vi "教導.vi"() -> ()   [LabVIEW 2015]
panel:
  out "密碼正確":bool
  in  "02A-5 Home Flag":bool
  out "Home TimeOut 2":dbl format="%.2f"
  in  "Home TimeOut In 2":dbl=30000.0 format="%#_13g"
  out "單軸復歸進行 2":bool
  out "Home TimeOut":dbl format="%.2f"
  in  "Home TimeOut In":dbl=30000.0 format="%#_13g"
  out "單軸復歸進行":bool
  out "存檔":bool
  in  "Recipe Ring":u8(ring) items=["abc.ini", "LeTV.ini", "小米.ini"]
  in  "Jog_Speed":i32
  in  "Jog Ring":u16(ring) items=["距離移動", "連續移動"]
  in  "Step Ring":u16(ring) items=["0.001 mm", "0.01 mm", "0.1 mm", "1 mm"]
  out "Tab 機構部件":T1(tab)
  out "Tab 設定位置入Tray站":enum32{"取Tray馬達", "收Tray馬達"}(tab) caption="Tab 設定位置"
  in  "入Tray站_分Tray位":dbl=100.0 caption="分Tray位" min=100.0 max=115.0
  in  "入Tray站_取Tray位":dbl=120.0 caption="取Tray位" min=115.0 max=125.0
  in  "入Tray站_待Tray位":dbl caption="待Tray位" min=0.0 max=5.0
  in  "Save_入Tray站_取Tray馬達":bool
  in  "入Tray站_收Tray位":dbl caption="收Tray上升距離" min=0.0 max=40.0
  in  "Save_入Tray站_收Tray馬達":bool
  in  "JOG_Up":bool
  in  "JOG_Down":bool
  in  "馬達選擇":u32(ring) items=["取Tray馬達", "收Tray馬達"]
  out "Tab 設定位置入料站":enum32{"等待位", "取料位", "放料位", "拍照位"}(tab) caption="Tab 設定位置"
  in  "JOG_Up 2":bool
  in  "JOG_Down 2":bool
  in  "JOG_R 2":bool
  in  "JOG_L 2":bool
  in  "點位選擇02A":u32(ring) items=["等待位", "取料位", "放料位", "拍照位"]
  in  "小Y":bool caption="Y¶b(¤pY)"
  in  "JOG_Down 2b 2":bool
  in  "JOG_Up 2b 2":bool
  in  "JOG_C02-":bool
  in  "JOG_C02+":bool
  in  "JOG_C01-":bool
  in  "JOG_C01+":bool
  in  "JOG_R 2b2":bool
  in  "JOG_L 2b2":bool
  out "Tab 設定位置入料站02B":enum32{"取料位", "安全位", "NG位", "拍照位", "放料位"}(tab) caption="Tab 設定位置"
  in  "JOG_Up 2b":bool
  in  "JOG_Down 2b":bool
  in  "JOG_R 2b1":bool
  in  "JOG_L 2b1":bool
  in  "點位選擇02B":u32(ring) items=["取料位", "安全位", "NG位", "拍照位", "放料位", "", ""]
  out "Tab 設定位置Ag站":enum32{"清潔位"}(tab) caption="Tab 設定位置"
  in  "JOG_Up 4":bool
  in  "JOG_Down 4":bool
  in  "JOG_R 4":bool
  in  "JOG_L 4":bool
  in  "點位選擇04":u32(ring) items=["清潔位", "取料位", "放料位"]
  out "Tab 設定位置UV站":enum32{"清潔位", "點膠位"}(tab) caption="Tab 設定位置"
  in  "JOG_Up 5":bool
  in  "JOG_Down 5":bool
  in  "JOG_R 5":bool
  in  "JOG_L 5":bool
  in  "點位選擇05":u32(ring) items=["清潔位", "點膠位", "放料位"]
  in  "JOG_旋轉 +":bool
  in  "JOG_旋轉 -":bool
  out "Tab 設定位置\n出料站":enum32{"等待位", "取料位", "放料位"}(tab) caption="Tab 設定位置"
  in  "JOG_Up 9":bool
  in  "JOG_Down 9":bool
  in  "JOG_R 9":bool
  in  "JOG_L 9":bool
  in  "點位選擇09":u32(ring) items=["等待位", "取料位", "放料位"]
  out "Tab 設定位置出Tray站":enum32{"取Tray馬達", "收Tray馬達"}(tab) caption="Tab 設定位置"
  in  "JOG_Up 10":bool
  in  "JOG_Down 10":bool
  out "出Tray站_馬達位置":dbl caption="馬達位置"
  in  "馬達選擇10":u32(ring) items=["取Tray馬達", "收Tray馬達"]
  in  "機構部件":T2(ring)
  in  "Exit":bool
  # "教導"
  # "馬達移動"
  # "mm/s"
  # "現在位置(mm)"
  # "JOG"
  # "設定位置(mm)"
  # "設定位置(mm)"
  # "現在位置(mm)"
  # "JOG"
  # "設定位置(mm)"
  # "設定位置(mm)"
  # "設定位置(mm)"
  # "設定位置(mm)"
  # "現在位置(mm)"
  # "JOG"
  # "設定位置(mm)"
  # "設定位置(mm)"
  # "設定位置(mm)"
  # "設定位置(mm)"
  # "設定位置(mm)"
  # "現在位置(mm)"
  # "JOG"
  # "設定位置(mm)"
  # "現在位置(mm)"
  # "JOG"
  # "設定位置(mm)"
  # "設定位置(mm)"
  # "現在位置(mm)"
  # "JOG"
  # "設定位置(mm)"
  # "設定位置(mm)"
  # "設定位置(mm)"
  # "現在位置(mm)"
  # "JOG"
  # "設定位置(mm)"
  # "設定位置(mm)"
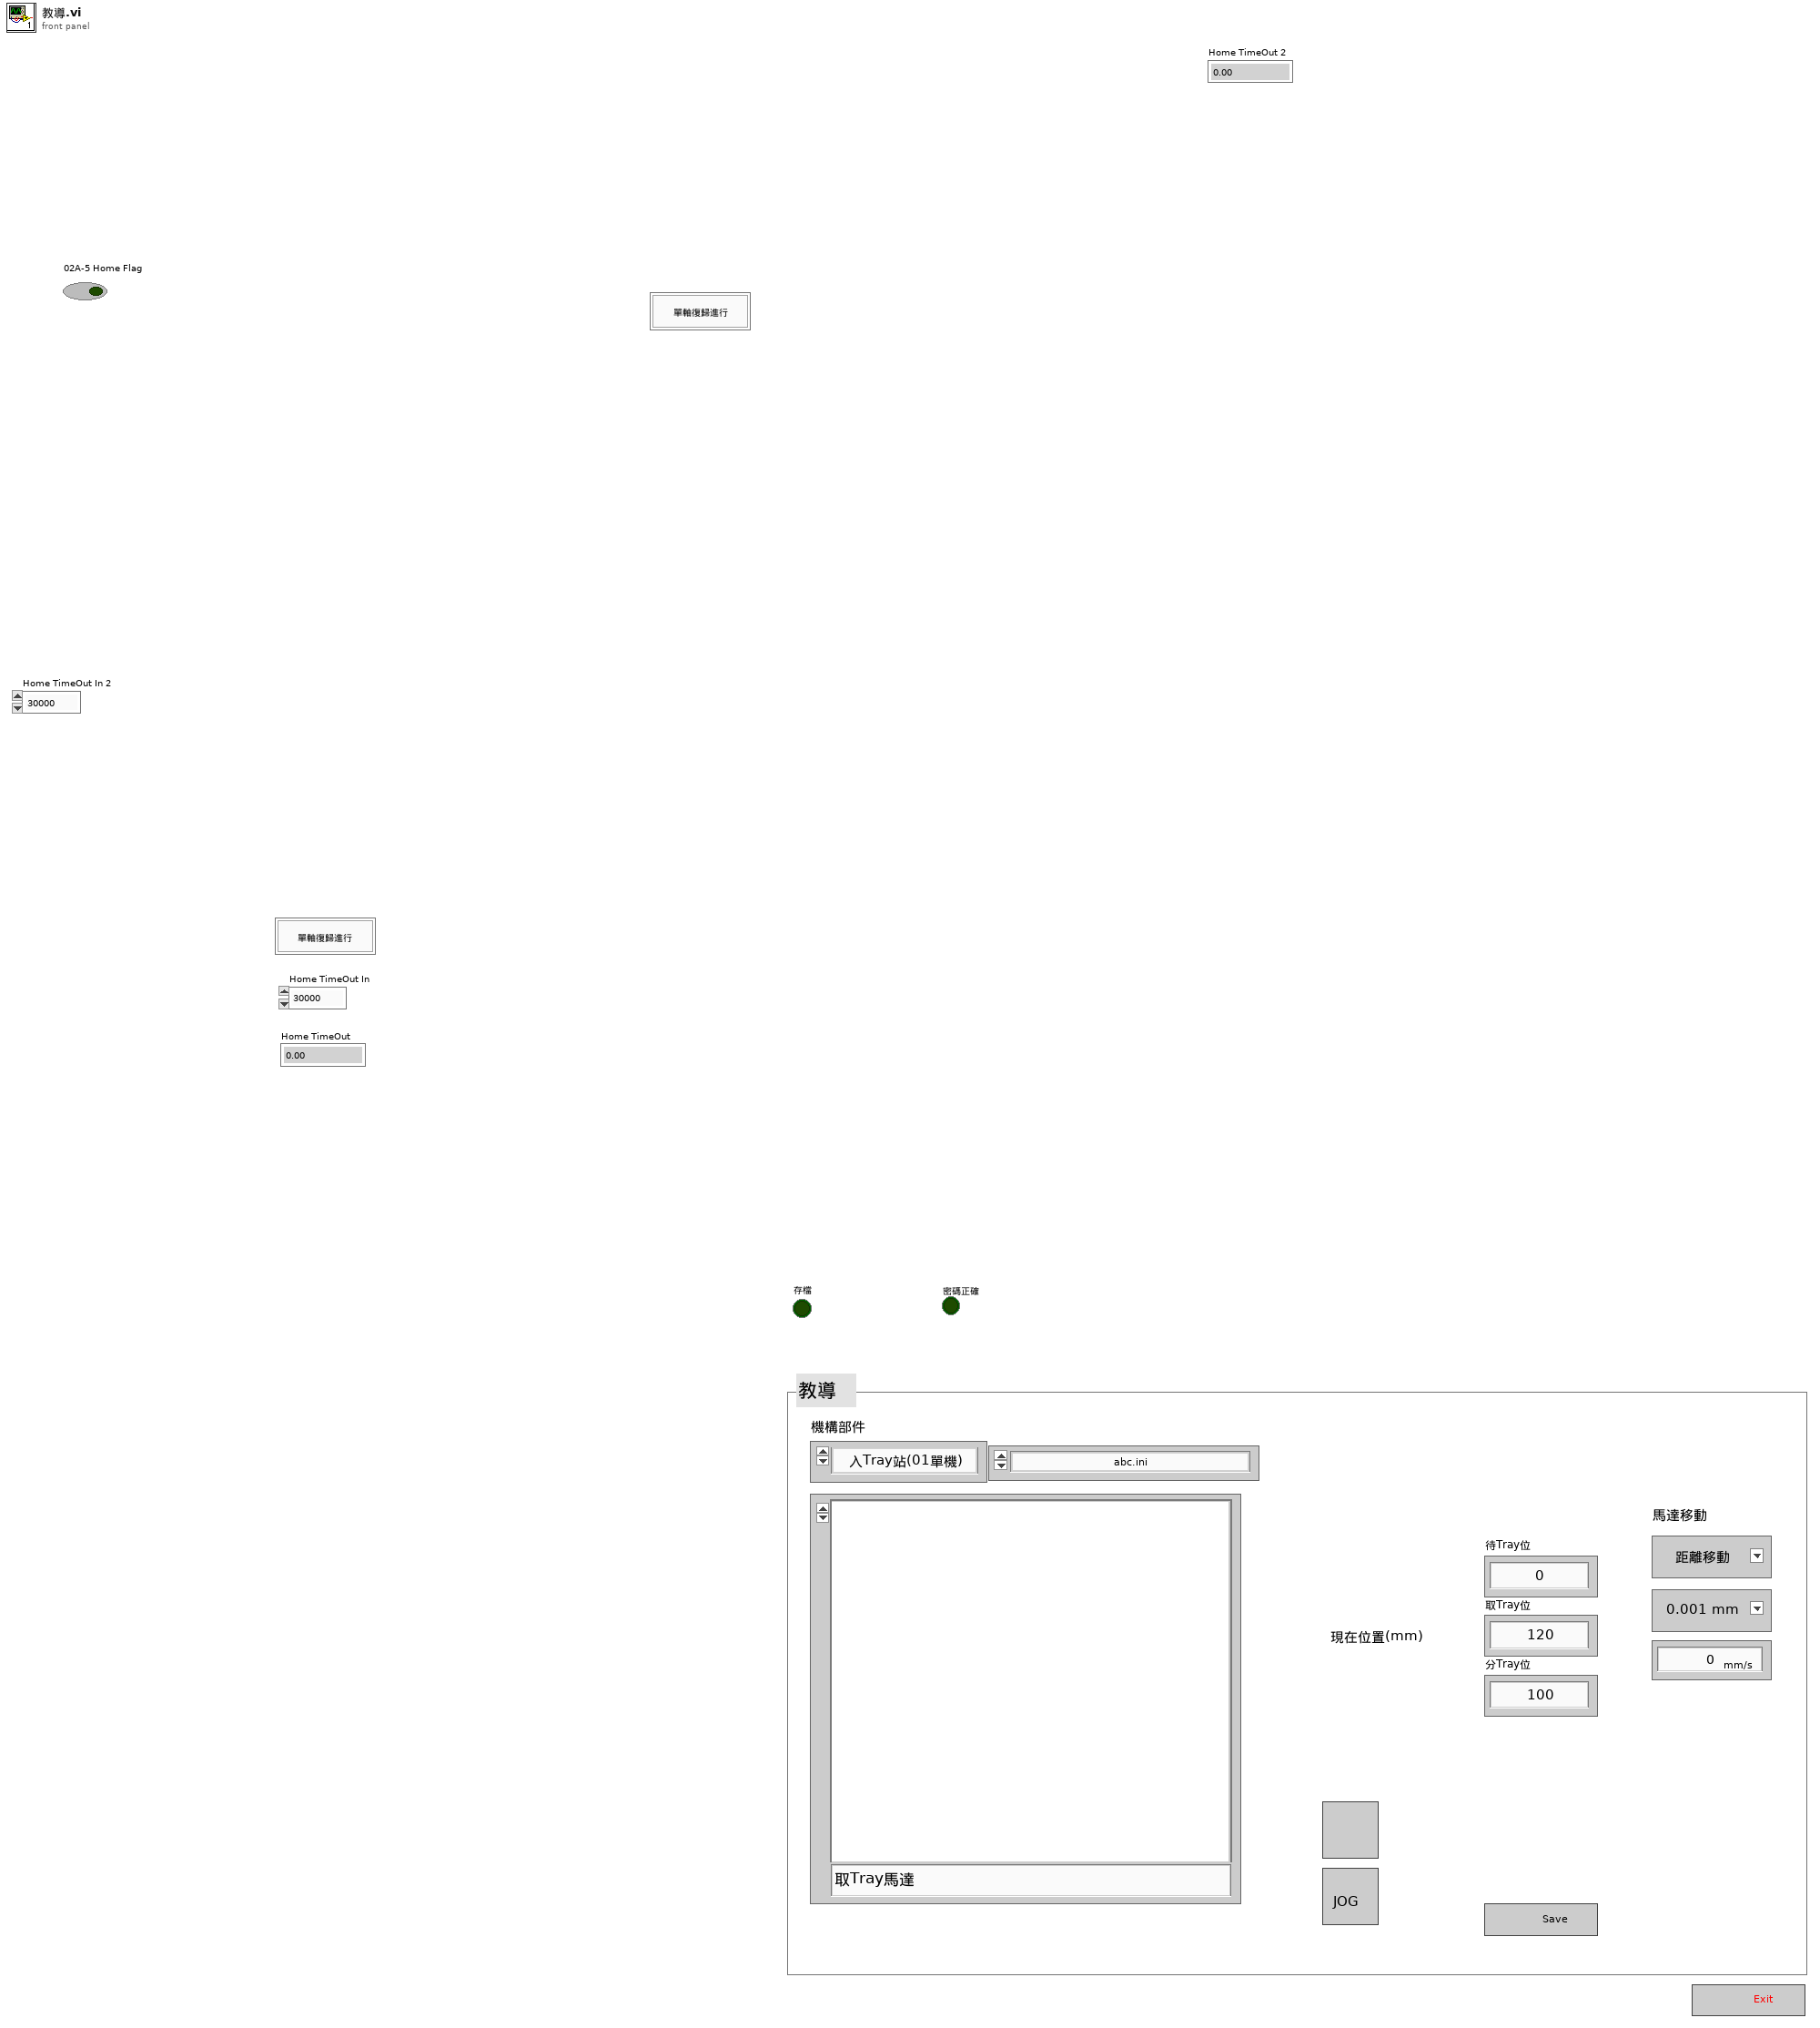
[diagram p1: front panel]
types:
  T1 = enum32{"入Tray端(01單機)", "入料端(02單機) ", "對位端(02單機)", "Ag端(04單機)", "UV端(05單機)", "出料端(09單機)", "出Tray端(10單機)"}
  T2 = enum32{"入Tray站(01單機)", "入料站(02單機)", "對位站(02單機)", "Ag站(04單機)", "UV站(05單機)", "出料站(09單機)", "出Tray站(10單機)"}
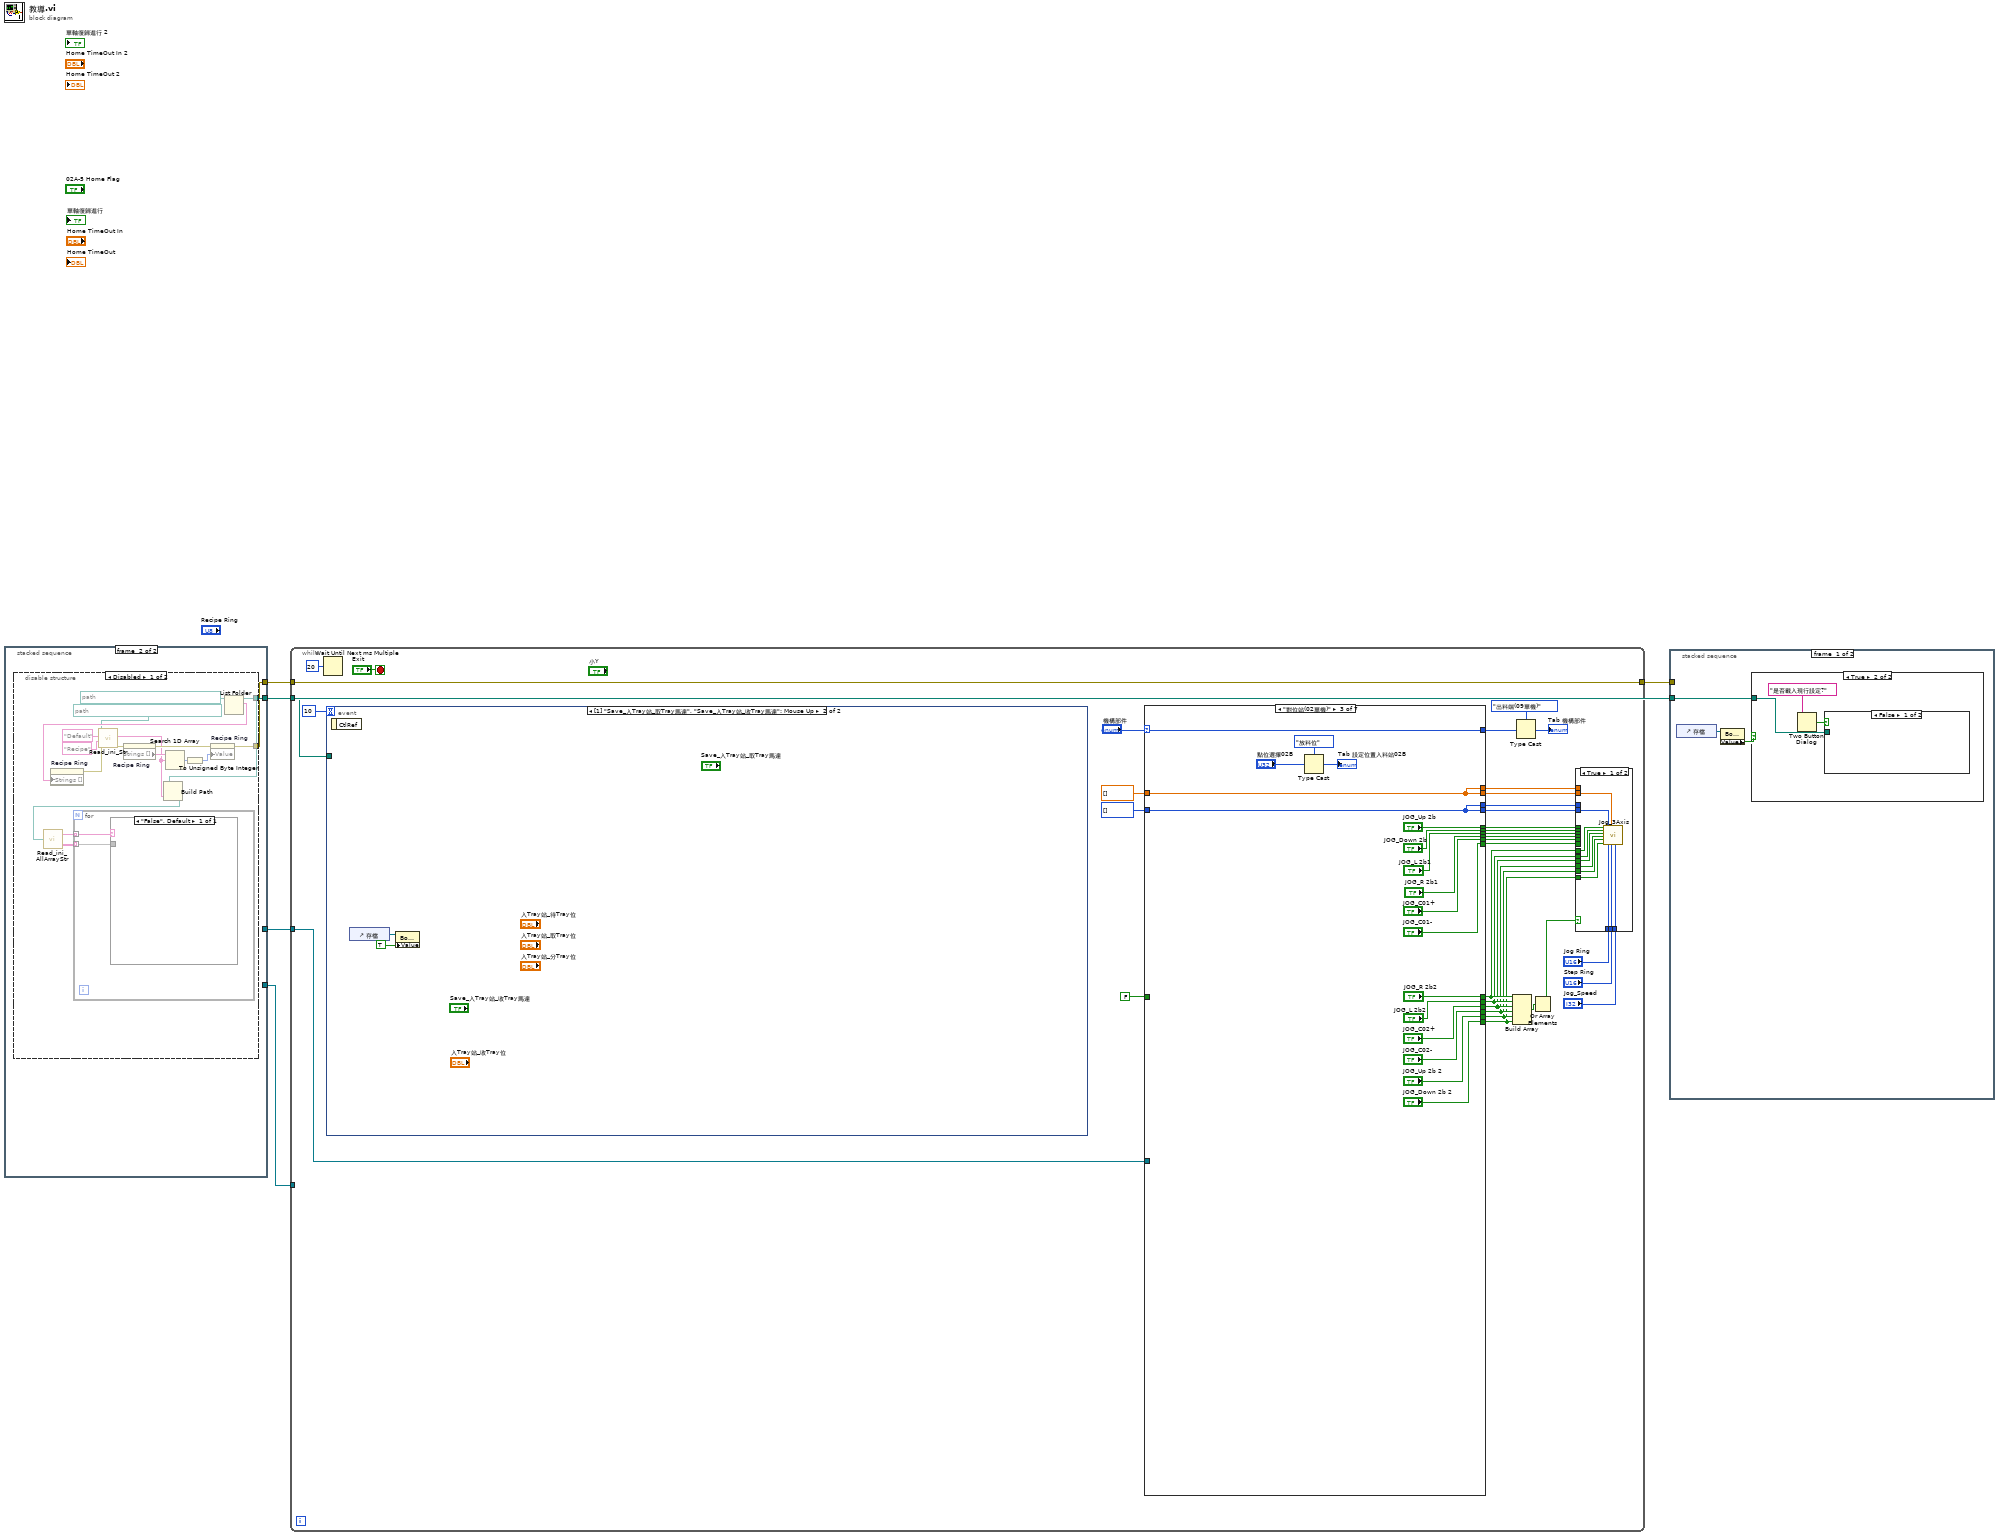
[diagram p0: block diagram]
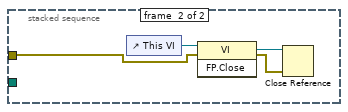
[diagram p4: hidden frame]
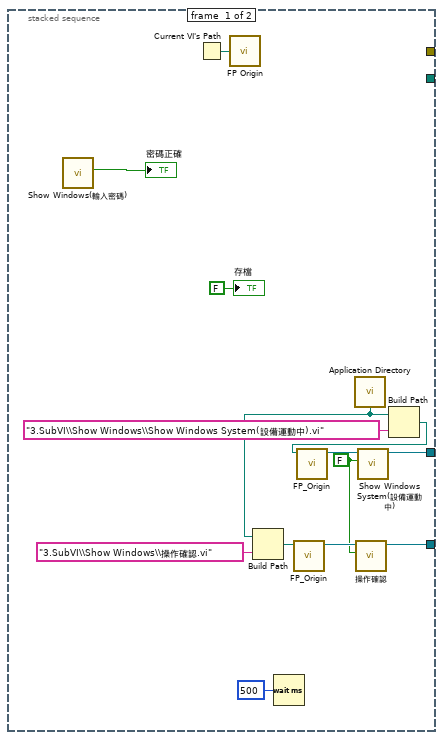
[diagram p5: hidden frame]
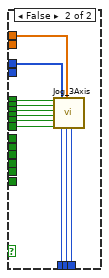
[diagram p7: hidden frame]
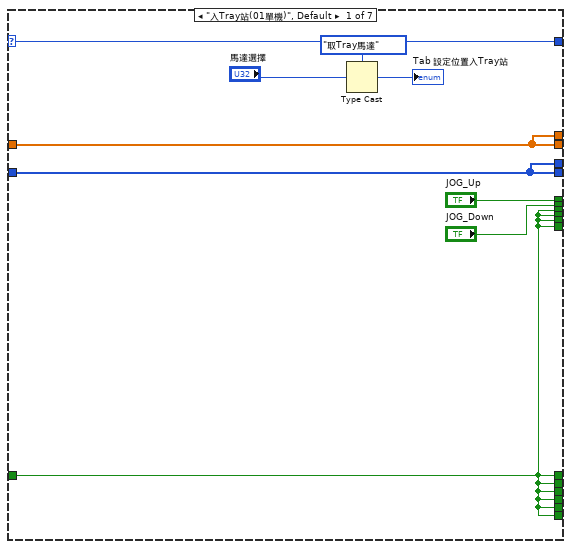
[diagram p8: hidden frame]
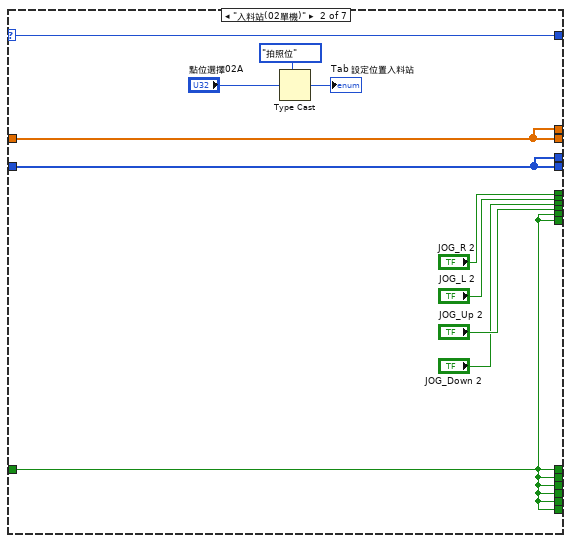
[diagram p9: hidden frame]
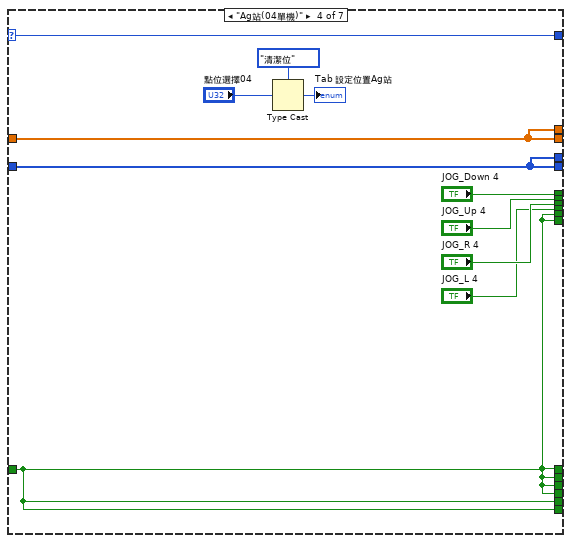
[diagram p10: hidden frame]
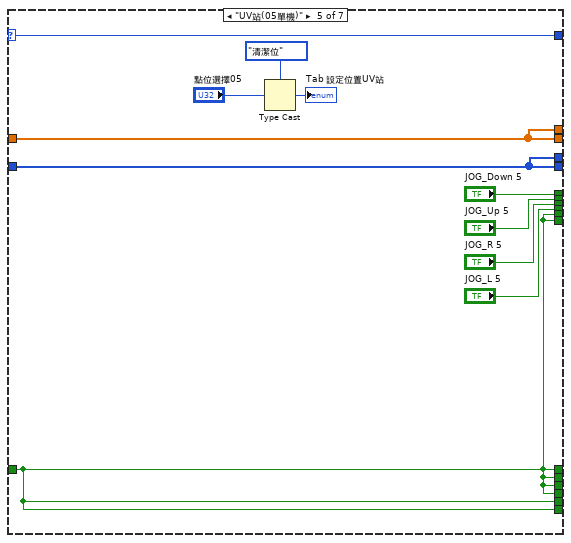
[diagram p11: hidden frame]
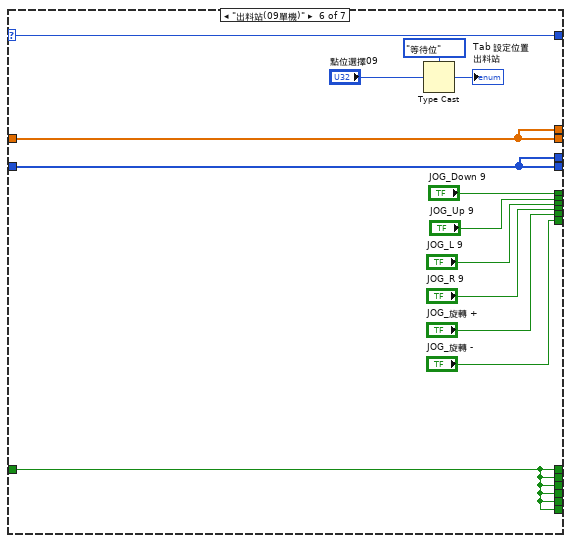
[diagram p12: hidden frame]
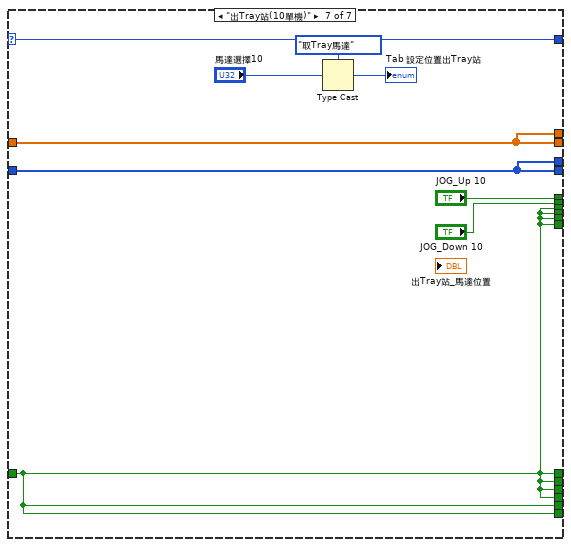
[diagram p13: hidden frame]
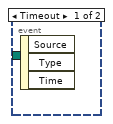
[diagram p14: hidden frame]
diagram:
  n1 = stacked-sequence {
    tunnel: [_ w20] -> w2
    tunnel: [_ w21] -> w4
    tunnel: [w14 _] -> w3
    tunnel: [w8 _] -> w1
    frame #0 {
      w10 = FALSE ("Show")
      n2 = call "Show Windows(輸入密碼).vi"() -> ("密碼正確"=→"密碼正確":bool)  [unwired: 10 in, 1 out]
      n3 = Current VI's Path() -> (path=w19:path)
      n4 = call "FP Origin.vi"("vi path"=w19) -> ()  [unwired: 1 out]
      n5 = Wait (ms)(milliseconds to wait=u32 500) -> ()  [unwired: 1 out]
      n6 = call <vilib>:"Application Directory.vi"() -> ("Application Directory"=w9:path)
      n7 = Build Path(base path=w9, name or relative path="3.SubVI\\Show Windows\\操作確認.vi") -> (appended path=w11:path)
      n8 = call "FP_Origin.vi"("VI.Path"=w11) -> ("VI Reference"=w13:refnum<vi>)  [unwired: 9 in, 1 out]
      n9 = call "操作確認.vi"("Show"=w10, "vi reference in"=w13) -> ("vi reference out"=w8:refnum<vi>)  [unwired: 6 in, 2 out]
      n10 = Build Path(base path=w9, name or relative path="3.SubVI\\Show Windows\\Show Windows System(設備運動中).vi") -> (appended path=w17:path)
      n11 = call "FP_Origin.vi"("VI.Path"=w17) -> ("VI Reference"=w16:refnum<vi>)  [unwired: 9 in, 1 out]
      n12 = call "Show Windows System(設備運動中).vi"("Show"=w10, "vi reference in"=w16) -> ("vi reference out"=w14:refnum<vi>)  [unwired: 8 in, 1 out]
      "存檔" <- FALSE ("存檔")
    }
    frame #1 {
      n13 = disable-structure shown="Disabled" {
        disable-tunnel: [w26 _] -> w21
        disable-tunnel: [w22 _] -> w20
        frame Disabled {
          n14 = List Folder(path=path "D:/半自動電檢機 Data/Recipe/Position" ("configuration file path")) -> (path out=w26:path, filenames=w32:string[])  [unwired: 3 in, 2 out]
          n15 = property on="Recipe Ring" class="Ring (strict)"("Strings []"=w32) -> (error out=w33:errorcluster)  [unwired: 2 in, 1 out]
          n16 = call "Read_ini_Str.vi"("error in (no error)"=w33, "key"="Recipe", "section"="Default", "configuration file path"=path "D:/半自動電檢機 Data/Recipe/Default.ini") -> ("error out"=w34:errorcluster, "value"=w25:string)  [unwired: 6 in]
          n17 = property on="Recipe Ring" class="Ring (strict)"(error in=w34) -> (error out=w36:errorcluster, "Strings []"=w35:string[])  [unwired: 1 in, 1 out]
          n18 = Build Path(base path=w26, name or relative path=w25) -> (appended path=w24:path)
          n19 = call "Read_ini_AllArrayStr.vi"("configuration file path"=w24) -> ("Section"=w37:string[], "Value"=w38:string[][])
          n20 = for {
            tunnel: w37 -> [w40] mode=indexing
            tunnel: w38 -> [w39] mode=indexing
            n21 = case shown="\"False\", Default" w40 {
              tunnel: w39 -> [_]
              frame "False", Default {
              }
            }
          }
          n22 = Search 1D Array(1D array=w35, element=w25) -> (index of element=w28:i32)  [unwired: 1 in]
          n23 = To Unsigned Byte Integer(number=w28) -> (unsigned 8bit integer=w23:u8)
          n24 = property on="Recipe Ring" class="Ring (strict)"(error in=w36, "Value"=w23) -> (error out=w22:errorcluster)  [unwired: 1 in, 1 out]
        }
        frame Enabled {
        }
      }
    }
  }
  n25 = while {
    tunnel: w2 -> [w71]
    tunnel: [w71] -> w5
    tunnel: w4 -> [w66]
    tunnel: w3 -> [w41]
    tunnel: w1 -> [_]
    stop <- "Exit" stop-if-true
    n26 = Wait Until Next ms Multiple(millisecond multiple=u32 20) -> ()  [unwired: 1 out]
    n27 = event shown="[1] \"Save_入Tray站_取Tray馬達\", \"Save_入Tray站_收Tray馬達\": Mouse Up" {
      selector: _ -> [_ _]
      dyn-events: _ -> [_ _]
      timeout: 10 -> [_ _]
      tunnel: w66 -> [_ _]
      event Timeout {
        n28 = event-data() -> ()  [unwired: 1 in, 3 out]
      }
      event "Save_入Tray站_取Tray馬達", "Save_入Tray站_收Tray馬達": Mouse Up {
        n29 = event-data() -> ()  [unwired: 1 in, 1 out]
        n30 = control-ref of="存檔"() -> (w179:refnum<vi>)
        n31 = property class="Bool (strict)"(reference=w179, "Value"=TRUE) -> ()  [unwired: 1 in, 2 out]
      }
    }
    n32 = case shown="\"對位站(02單機)\"" "機構部件" {
      selector: "機構部件" -> [w105 w116 w119 w145 w156 w169 w178]
      tunnel: [w105 w116 w119 w145 w156 w169 w178] -> w69
      tunnel: ["JOG_Up" "JOG_R 2" "JOG_Up 2b" "JOG_Down 4" "JOG_Down 5" "JOG_Down 9" "JOG_Up 10"] -> w65
      tunnel: ["JOG_Down" "JOG_L 2" "JOG_Down 2b" "JOG_Up 4" "JOG_Up 5" "JOG_Up 9" "JOG_Down 10"] -> w64
      tunnel: [w99 w106 w117 w136 w146 w158 w170] -> w63
      tunnel: [w98 w107 w118 w135 w147 w159 w171] -> w62
      tunnel: [w97 "JOG_Down 2" "JOG_L 2b1" "JOG_R 4" "JOG_R 5" "JOG_L 9" w173] -> w58
      tunnel: [w97 "JOG_Up 2" "JOG_R 2b1" "JOG_L 4" "JOG_L 5" "JOG_R 9" w173] -> w57
      tunnel: [w97 w108 "JOG_C01+" w137 w154 "JOG_旋轉 +" w173] -> w56
      tunnel: [w97 w108 "JOG_C01-" w137 w154 "JOG_旋轉 -" w173] -> w55
      tunnel: [w97 w108 "JOG_R 2b2" w137 w154 w157 w173] -> w47
      tunnel: [w97 w108 "JOG_L 2b2" w137 w154 w157 w173] -> w46
      tunnel: [w97 w108 "JOG_C02+" w137 w154 w157 w173] -> w45
      tunnel: [w97 w108 "JOG_C02-" w137 w154 w157 w173] -> w44
      tunnel: [w98 w107 w118 w135 w147 w159 w171] -> w52
      tunnel: [w99 w106 w117 w136 w146 w158 w170] -> w51
      tunnel: dbl[] [] ("ResolutionArray") -> [w98 w107 w118 w135 w147 w159 w171]
      tunnel: i32[] [] ("AxisArray") -> [w99 w106 w117 w136 w146 w158 w170]
      tunnel: FALSE ("JOG_L 2b2") -> [w97 w108 _ w137 w154 w157 w173]
      tunnel: [w97 w108 "JOG_Up 2b 2" w137 w154 w157 w173] -> w43
      tunnel: [w97 w108 "JOG_Down 2b 2" w137 w154 w157 w173] -> w42
      tunnel: w41 -> [_ _ _ _ _ _ _]
      frame "入Tray站(01單機)", Default {
        n33 = Type Cast(type=enum32{"取Tray馬達", "收Tray馬達"}."取Tray馬達" ("Tab 設定位置"), x="馬達選擇") -> (*(type *) &x=→"Tab 設定位置入Tray站":enum32{"取Tray馬達", "收Tray馬達"})
      }
      frame "入料站(02單機)" {
        n34 = Type Cast(type=enum32{"等待位", "取料位", "放料位", "拍照位"}."拍照位" ("Tab 設定位置入料站"), x="點位選擇02A") -> (*(type *) &x=→"Tab 設定位置入料站":enum32{"等待位", "取料位", "放料位", "拍照位"})
      }
      frame "對位站(02單機)" {
        n35 = Type Cast(type=enum32{"取料位", "安全位", "NG位", "拍照位", "放料位"}."放料位" ("Tab 設定位置\n入料站02B"), x="點位選擇02B") -> (*(type *) &x=→"Tab 設定位置入料站02B":enum32{"取料位", "安全位", "NG位", "拍照位", "放料位"})
      }
      frame "Ag站(04單機)" {
        n36 = Type Cast(type=enum32{"清潔位"}."清潔位" ("Tab 設定位置\nAg站"), x="點位選擇04") -> (*(type *) &x=→"Tab 設定位置Ag站":enum32{"清潔位"})
      }
      frame "UV站(05單機)" {
        n37 = Type Cast(type=enum32{"清潔位", "點膠位"}."清潔位" ("Tab 設定位置UV站"), x="點位選擇05") -> (*(type *) &x=→"Tab 設定位置UV站":enum32{"清潔位", "點膠位"})
      }
      frame "出料站(09單機)" {
        n38 = Type Cast(type=enum32{"等待位", "取料位", "放料位"}."等待位" ("Tab 設定位置\n入料站"), x="點位選擇09") -> (*(type *) &x=→"Tab 設定位置\n出料站":enum32{"等待位", "取料位", "放料位"})
      }
      frame "出Tray站(10單機)" {
        n39 = Type Cast(type=enum32{"取Tray馬達", "收Tray馬達"}."取Tray馬達" ("Tab 設定位置"), x="馬達選擇10") -> (*(type *) &x=→"Tab 設定位置出Tray站":enum32{"取Tray馬達", "收Tray馬達"})
      }
    }
    n40 = Build Array(w47, w46, w45, w44, w43, w42) -> (w54:bool[])
    n41 = Type Cast(type=T1."出料端(09單機)" ("Tab 機構部件"), x=w69) -> (*(type *) &x=→"Tab 機構部件":T1)
    n42 = Or Array Elements(Boolean array=w54) -> (logical OR=w53:bool)
    n43 = case shown="True" w53 {
      tunnel: w65 -> [_ w96]
      tunnel: w64 -> [_ w95]
      tunnel: w63 -> [_ w94]
      tunnel: w62 -> [_ w93]
      tunnel: "Jog Ring" -> [w85 w92]
      tunnel: "Step Ring" -> [w84 w91]
      tunnel: "Jog_Speed" -> [w75 w90]
      tunnel: w58 -> [_ w89]
      tunnel: w57 -> [_ w88]
      tunnel: w56 -> [_ w87]
      tunnel: w55 -> [_ w86]
      tunnel: w52 -> [w83 _]
      tunnel: w51 -> [w82 _]
      tunnel: w47 -> [w81 _]
      tunnel: w46 -> [w80 _]
      tunnel: w45 -> [w79 _]
      tunnel: w44 -> [w78 _]
      tunnel: w43 -> [w77 _]
      tunnel: w42 -> [w76 _]
      frame True {
        n44 = call "Jog_3Axis.vi"("JOG_Up"=w81, "JOG_Down"=w80, "JOG_R"=w79, "JOG_L"=w78, "JOG_C+"=w77, "JOG_C-"=w76, "AxisArray"=w82, "Jog Ring"=w85, "ResolutionArray"=w83, "Step Ring"=w84, "Jog_Speed"=w75) -> ()  [unwired: 9 in]
      }
      frame False {
        n45 = call "Jog_3Axis.vi"("JOG_Up"=w96, "JOG_Down"=w95, "JOG_R"=w89, "JOG_L"=w88, "JOG_C+"=w87, "JOG_C-"=w86, "AxisArray"=w94, "Jog Ring"=w92, "ResolutionArray"=w93, "Step Ring"=w91, "Jog_Speed"=w90) -> ()  [unwired: 9 in]
      }
    }
  }
  n46 = stacked-sequence {
    tunnel: w5 -> [_ w190]
    tunnel: w4 -> [w183 _]
    frame #0 {
      n47 = control-ref of="存檔"() -> (w182:refnum<vi>)
      n48 = property class="Bool (strict)"(reference=w182) -> ("Value"=w181:bool)  [unwired: 1 in, 2 out]
      n49 = case shown="True" w181 {
        tunnel: w183 -> [_ w184]
        frame False {
        }
        frame True {
          n50 = Two Button Dialog(message="是否載入現行設定?") -> (T button?=w185:bool)  [unwired: 2 in]
          n51 = case shown="False" w185 {
            tunnel: w184 -> [_ _]
            frame False {
            }
            frame True {
            }
          }
        }
      }
    }
    frame #1 {
      n52 = control-ref of="This VI"() -> (w189:refnum<vi>)
      n53 = invoke class="VI" method="FP.Close"(reference=w189, error in=w190) -> (reference out=w188:refnum<vi>, error out=w187:errorcluster)  [unwired: 1 in, 1 out]
      n54 = Close Reference(reference=w188, error in (no error)=w187) -> ()  [unwired: 1 out]
    }
  }
